vi "Add File Name on PDF.vi"(11 "error in (no error)":errorcluster) -> (6 "Path":path, 15 "error out":errorcluster)   [LabVIEW 2019]
doc: "Location: at the end of the report generation.\n\nThis can only be followed by \"Print PDF.vi\" and \"Dispose references.vi\".\n\nVersion 1.0\nDeveloped by Jean-Marc Simard\nCopyright © 2010, Exaprom Inc.\nAll rights reserved.\nLicense: BSD\n\nWith iTextSharp Library\n(http://itextsharp.sourceforge.net)"
uses:
  <userlib>/Exaprom PDF/LV Class/Header and Footer Class/VIs/Controls/Header Footer [ ] V2.ctl
  <userlib>/Exaprom PDF/LV Class/Header and Footer Class/VIs/Controls/Header Footer cluster V2.ctl
  <userlib>/Exaprom PDF/Controls/Header, Footer and Watermark Controls/Header or Footer.ctl
  <userlib>/Exaprom PDF/Controls/Header, Footer and Watermark Controls/Header Footer Type.ctl
  <userlib>/Exaprom PDF/Controls/Header, Footer and Watermark Controls/Header footer horiz alignment.ctl
  <userlib>/Exaprom PDF/Controls/Table Controls/Cell Vertical alignment.ctl
  <userlib>/Exaprom PDF/Controls/Text Controls/Line spacing.ctl
  <userlib>/Exaprom PDF/Controls/Header, Footer and Watermark Controls/Page number.ctl
  <userlib>/Exaprom PDF/Controls/Font Controls/Font complete cluster horizontal.ctl
  <userlib>/Exaprom PDF/Controls/Font Controls/Font size.ctl
  <userlib>/Exaprom PDF/Controls/Font Controls/Font color.ctl
  <userlib>/Exaprom PDF/Controls/Font Controls/Type and encoding.ctl
  <userlib>/Exaprom PDF/Controls/Text Controls/Unicode/Type and run direction.ctl
  C:/Program Files/National Instruments/LabVIEW 2019/user.lib/Exaprom PDF/DLL/itextsharp.dll
  DLL/itextsharp.dll
  <userlib>/Exaprom PDF/Controls/Header, Footer and Watermark Controls/Header Footer Line.ctl
  <userlib>/Exaprom PDF/Controls/Page Controls/Page dimensions.ctl
  <userlib>/Exaprom PDF/Controls/Page Controls/Page size.ctl
  <userlib>/Exaprom PDF/Controls/Page Controls/Page Orientation.ctl
panel:
  in  "Header or Footer [ ]":T1
  in  "Path 2":path
  # "X"
  # "Y"
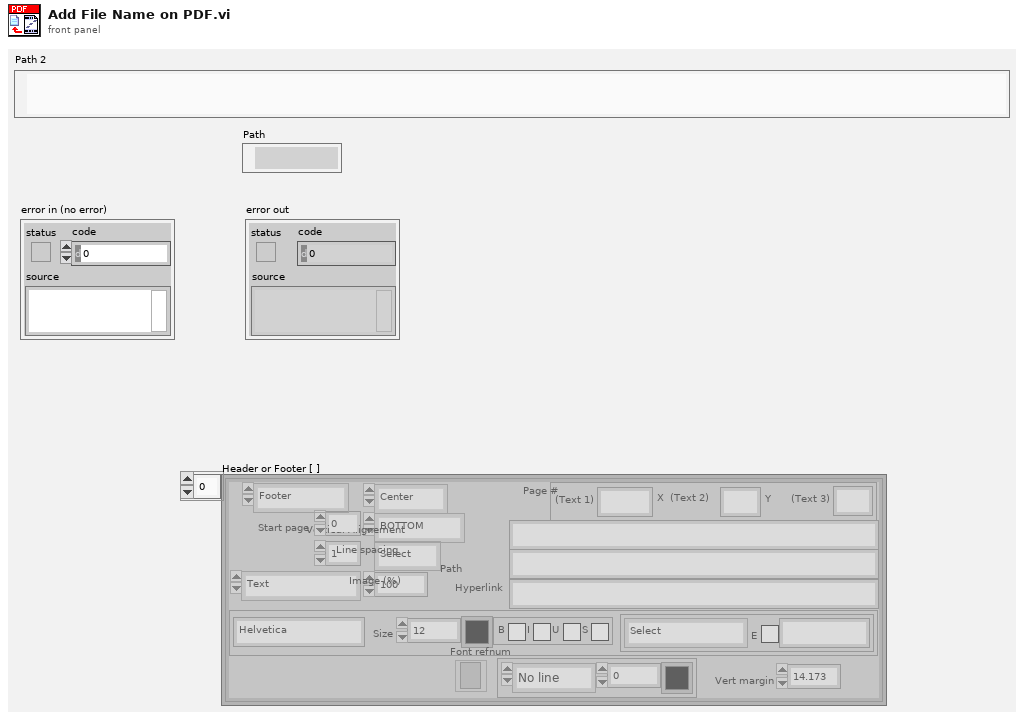
[diagram p1: front panel]
types:
  T1 = typedef "Header Footer [ ] V2.ctl" = T2[]
  T2 = typedef "Header Footer cluster V2.ctl" = cluster{"Header or Footer":T3, "Start page":i32, "Start with #":i32, "Type":T4, "Alignment":T5, "Vertical Alignement":T6, "Line spacing":T7, "Image (%)":sgl, "Page #":T8, "Text":string, "Path":string, "Font":T9, "Font refnum":refnum<k24>, "Line":cluster{"Line":T14, "Thickness (points)":sgl, "Colour":T11}, "Vert margin":dbl, "Hyperlink":string}
  T3 = typedef "Header or Footer.ctl" = enum16{"Header", "Footer"}
  T4 = typedef "Header Footer Type.ctl" = enum16{"Select", "Text", "Text + hyperlink", "Page number", "Image", "Image + hyperlink"}
  T5 = typedef "Header footer horiz alignment.ctl" = enum16{"Left", "Center", "Right"}
  T6 = typedef "Cell Vertical alignment.ctl" = enum16{"TOP", "MIDDLE", "BOTTOM"}
  T7 = typedef "Line spacing.ctl" = enum16{"Select", "1.0", "1.5", "2.0"}
  T8 = typedef "Page number.ctl" = cluster{"Text 1":string, "Text 2":string, "Text 3":string}
  T9 = typedef "Font complete cluster horizontal.ctl" = cluster{"Name":string, "Size":T10, "Color":T11, "Style":cluster{"Bold":bool, "Italic":bool, "Underline":bool, "Strikeout":bool}, "Type":T12}
  T10 = typedef "Font size.ctl" = sgl
  T11 = typedef "Font color.ctl" = u32
  T12 = typedef "Type and encoding.ctl" = cluster{"Type&direction":T13, "Embedded":bool, "Encoding":string}
  T13 = typedef "Type and run direction.ctl" = enum16{"Select", "ASCII", "UTF-16", "UTF-16 (default)", "UTF-16 (LTR)", "UTF-16 (RTL)"}
  T14 = typedef "Header Footer Line.ctl" = enum16{"No line", "Horizontal line"}
  T15 = typedef "Page dimensions.ctl" = cluster{"Start at page":i32, "Page Size":T16, "Orientation":T17, "widht":sgl, "height":sgl, "Margin left":sgl, "Margin right":sgl, "Margin top":sgl, "Margin bottom":sgl, "X0":sgl, "X1":sgl, "Y0":sgl, "Y1":sgl}
  T16 = typedef "Page size.ctl" = i32
  T17 = typedef "Page Orientation.ctl" = enum16{"Portrait", "Landscape"}
  T18 = typedef "Header Footer Complete Cluster.ctl" = cluster{"Table position":T19, "Header Footer Cluster with references [ ]":T20[]}
  T19 = typedef "Header or Footer Position.ctl" = cluster{"Vert margin":dbl, "FixedHeight":dbl, "Table X postion":dbl, "Table Y postion":dbl}
  T20 = typedef "Header Footer Cluster with references.ctl" = cluster{"Start page":i32, "Type":T4, "Start with #":i32, "Alignment":T5, "Vertical Alignement":T6, "Page #":T8, "Text":refnum<k24>, "Scaled Img":refnum<k24>, "PdfPCell":refnum<k24>, "PdfPTable":refnum<k24>, "Font Cluster":T9, "Font ":refnum<k24>, "Img (%)":sgl, "Line":cluster{"Line":T14, "Thickness (points)":sgl, "Colour":T11}, "Line spacing":T7}
  T21 = typedef "Watermark cluster2.ctl" = cluster{"Show? (F)":bool, "Type":enum16{"Image", "Text"}, "Opacity (%)":sgl, "Rotate(°)":sgl, "Position":cluster{"Position":T22, "X":sgl, "Y":sgl}, "Image path":path, "Scaled(%)":sgl, "Image refnum":refnum<k24>, "Text":string, "Font":cluster{"Name":string, "Size":T10, "Color":T11}, "Font refnum":refnum<k24>, "Alignment":T5, "Automatic":bool}
  T22 = typedef "Watermark Position.ctl" = enum16{"Absolute", "Center (page)", "Center (text section)"}
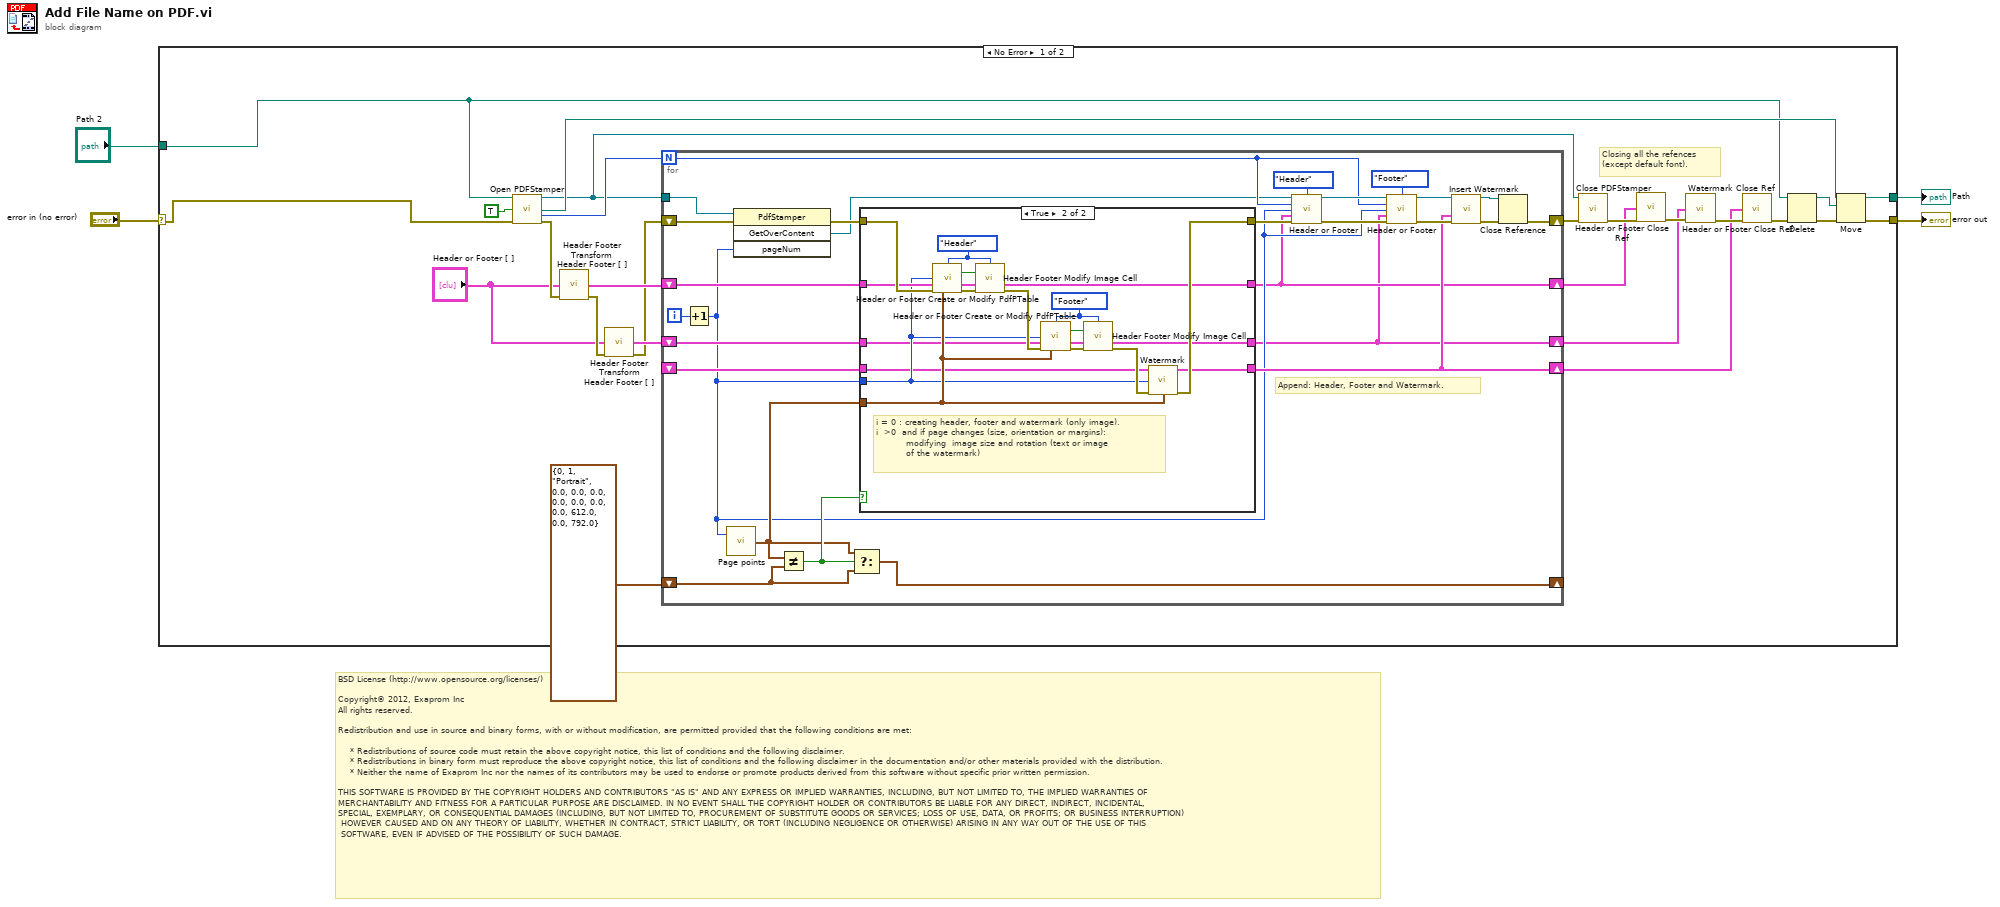
[diagram p0: block diagram]
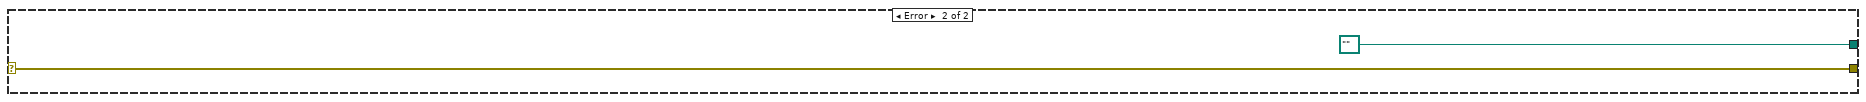
[diagram p3: hidden frame]
diagram:
  # "BSD License (http://www.opensource.org/licenses/)\n\nCopyright© 2012, Exaprom Inc\nAll rights reserved.\n\nRedistribution and use in source and binary forms, with or without modification, are permitted provided that the following conditions are met:\n\n    * Redistributions of source code must retain the above copyright notice, this list of conditions and the following disclaimer.\n    * Redistributions in binary form must reproduce the above copyright notice, this list of conditions and the following disclaimer in the documentation and/or other materials provided with the distribution.\n    * Neither the name of Exaprom Inc nor the names of its contributors may be used to endorse or promote products derived from this software without specific prior written permission.\n\nTHIS SOFTWARE IS PROVIDED BY THE COPYRIGHT HOLDERS AND CONTRIBUTORS \"AS IS\" AND ANY EXPRESS OR IMPLIED WARRANTIES, INCLUDING, BUT NOT LIMITED TO, THE IMPLIED WARRANTIES OF \nMERCHANTABILITY AND FITNESS FOR A PARTICULAR PURPOSE ARE DISCLAIMED. IN NO EVENT SHALL THE COPYRIGHT HOLDER OR CONTRIBUTORS BE LIABLE FOR ANY DIRECT, INDIRECT, INCIDENTAL,\nSPECIAL, EXEMPLARY, OR CONSEQUENTIAL DAMAGES (INCLUDING, BUT NOT LIMITED TO, PROCUREMENT OF SUBSTITUTE GOODS OR SERVICES; LOSS OF USE, DATA, OR PROFITS; OR BUSINESS INTERRUPTION)\n HOWEVER CAUSED AND ON ANY THEORY OF LIABILITY, WHETHER IN CONTRACT, STRICT LIABILITY, OR TORT (INCLUDING NEGLIGENCE OR OTHERWISE) ARISING IN ANY WAY OUT OF THE USE OF THIS\n SOFTWARE, EVEN IF ADVISED OF THE POSSIBILITY OF SUCH DAMAGE."
  n1 = case shown="No Error" "error in (no error)" {
    selector: "error in (no error)" -> [w6 w82]
    tunnel: [w8 w82] -> w4
    tunnel: [w29 path "" ("new path")] -> w2
    tunnel: "Path 2" -> [w7 _]
    frame No Error {
      # "Closing all the refences \n(except default font)."
      n2 = call <userlib>:"Open PDFStamper.vi"("PDF Path (original)"=w7, "RotateContents (F)"=TRUE, "error in (no error)"=w6) -> ("PDFStamper"=w19:refnum<k24>, "Temporary File Name"=w25:path, "NumberOfPages"=w27:i32, "error out"=w15:errorcluster)  [unwired: 4 in, 5 out]
      n3 = call <userlib>:"Header Footer Transform Header Footer [ ].vi"("Header or Footer [ ]"="Header or Footer [ ]", "error in (no error)"=w15) -> ("Header or Footer Complete Cluster"=w18:T18, "error out"=w16:errorcluster)  [unwired: 12 out]
      n4 = call <userlib>:"Header Footer Transform Header Footer [ ].vi"("Header or Footer [ ]"="Header or Footer [ ]", "error in (no error)"=w16) -> ("Header or Footer Complete Cluster"=w17:T18, "error out"=w14:errorcluster)  [unwired: 12 out]
      n5 = for {
        N: w27 -> [w45]
        tunnel: w19 -> [w50]
        shift-right: [w44] -> _
        shift-left: T15 {"Start at page"=0, "Page Size"=1, "Orientation"=enum."Portrait", "widht"=0.0, "height"=0.0, "Margin left"=0.0, "Margin right"=0.0, "Margin top"=0.0, "Margin bottom"=0.0, "X0"=0.0, "X1"=612.0, "Y0"=0.0, "Y1"=792.0} ("Page (points)") -> [w43]
        shift-right: [w38] -> w9
        shift-left: _ -> [w37]
        shift-right: [w36] -> w26
        shift-left: w14 -> [w51]
        shift-right: [w32] -> w13
        shift-left: w18 -> [w41]
        shift-right: [w31] -> w12
        shift-left: w17 -> [w39]
        i -> [w52]
        # "Append: Header, Footer and Watermark."
        n6 = Increment(x=w52) -> (x+1=w33:i32)
        n7 = call <userlib>:"Page points.vi"("pageNum"=w33) -> ("Page (points)"=w40:T15)  [unwired: 1 in]
        n8 = invoke class="PdfStamper" method="GetOverContent"(reference=w50, error in=w51, "pageNum"=w33) -> (error out=w55:errorcluster, "GetOverContent"=w30:refnum<k24>)  [unwired: 1 in, 2 out]
        n9 = Not Equal?(x=w40, y=w43) -> (x != y?=w42:bool)
        n10 = Select(t=w40, s=w42, f=w43) -> (s? t:f=w44:T15)
        n11 = case shown="True" w42 {
          tunnel: w41 -> [w59 w76]
          tunnel: w40 -> [_ w72]
          tunnel: w39 -> [w58 w63]
          tunnel: w55 -> [w57 w80]
          tunnel: [w57 w78] -> w56
          tunnel: w37 -> [w60 w68]
          tunnel: [w60 w73] -> w38
          tunnel: w33 -> [_ w71]
          tunnel: [w59 w65] -> w32
          tunnel: [w58 w64] -> w31
          frame False {
          }
          frame True {
            w69 = Header_or_Footer."Footer" ("Header or Footer")
            w70 = Header_or_Footer."Header" ("Header or Footer")
            # "i = 0 : creating header, footer and watermark (only image).\ni  >0  and if page changes (size, orientation or margins):\n          modifying  image size and rotation (text or image \n          of the watermark)"
            n12 = call <userlib>:"Header or Footer Create or Modify PdfPTable.vi"("Header or Footer"=w70, "pageNum"=w71, "Header Footer IN [ ]"=w76, "error in (no error)"=w80, "Page points"=w72) -> ("Modify Image Cell"=w62:bool, "Header Footer OUT [ ]"=w66:T18, "error out"=w75:errorcluster)  [unwired: 3 in, 5 out]
            n13 = call <userlib>:"Header Footer Modify Image Cell.vi"("Header or Footer"=w70, "Modify Image Cell"=w62, "Header or Footer Complete Cluster IN"=w66, "error in (no error)"=w75) -> ("Header or Footer Complete Cluster OUT"=w65:T18, "error out"=w77:errorcluster)  [unwired: 1 in, 9 out]
            n14 = call <userlib>:"Header or Footer Create or Modify PdfPTable.vi"("Header or Footer"=w69, "pageNum"=w71, "Header Footer IN [ ]"=w63, "error in (no error)"=w77, "Page points"=w72) -> ("Modify Image Cell"=w61:bool, "Header Footer OUT [ ]"=w67:T18, "error out"=w74:errorcluster)  [unwired: 3 in, 5 out]
            n15 = call <userlib>:"Header Footer Modify Image Cell.vi"("Header or Footer"=w69, "Modify Image Cell"=w61, "Header or Footer Complete Cluster IN"=w67, "error in (no error)"=w74) -> ("Header or Footer Complete Cluster OUT"=w64:T18, "error out"=w79:errorcluster)  [unwired: 1 in, 9 out]
            n16 = call <userlib>:"Watermark.vi"("Watermark IN"=w68, "pageNum"=w71, "error in (no error)"=w79, "Page dimensions"=w72) -> ("Watermark OUT"=w73:T21, "error out"=w78:errorcluster)  [unwired: 2 in, 8 out]
          }
        }
        n17 = call <userlib>:"Header or Footer.vi"("OverContent"=w30, "Header or Footer"=Header_or_Footer."Header", "NumberOfPages"=w45, "pageNum"=w33, "Header or Footer Complete Cluster"=w32, "error in (no error)"=w56) -> ("OverContent duplicate"=w53:refnum<k24>, "error out"=w54:errorcluster)  [unwired: 2 in, 6 out]
        n18 = call <userlib>:"Header or Footer.vi"("OverContent"=w53, "Header or Footer"=Header_or_Footer."Footer", "NumberOfPages"=w45, "pageNum"=w33, "Header or Footer Complete Cluster"=w31, "error in (no error)"=w54) -> ("OverContent duplicate"=w48:refnum<k24>, "error out"=w49:errorcluster)  [unwired: 1 in, 7 out]
        n19 = call <userlib>:"Insert Watermark.vi"("OverContent"=w48, "Watermark Cluster"=w38, "error in (no error)"=w49) -> ("OverContent duplicate"=w46:refnum<k24>, "error out"=w47:errorcluster)  [unwired: 3 in, 8 out]
        n20 = Close Reference(reference=w46, error in (no error)=w47) -> (error out=w36:errorcluster)
      }
      n21 = call <userlib>:"Close PDFStamper.vi"("PDFStamper"=w19, "error in (no error)"=w26) -> ("error out"=w21:errorcluster)  [unwired: 13 out]
      n22 = call <userlib>:"Header or Footer Close Ref.vi"("Header or Footer Complete Cluster"=w13, "error in (no error)"=w21) -> ("error out"=w20:errorcluster)  [unwired: 2 in, 11 out]
      n23 = call <userlib>:"Header or Footer Close Ref.vi"("Header or Footer Complete Cluster"=w12, "error in (no error)"=w20) -> ("error out"=w11:errorcluster)  [unwired: 1 in, 12 out]
      n24 = call <userlib>:"Watermark Close Ref.vi"("Watermark IN"=w9, "error in (no error)"=w11) -> ("error out"=w10:errorcluster)  [unwired: 1 in, 12 out]
      n25 = Delete(path (use dialog)=w7, error in=w10) -> (deleted path=w23:path, error out=w22:errorcluster)  [unwired: 4 out]
      n26 = Move(source path=w25, error in=w22, 10:w23) -> (error out=w8:errorcluster, 3:w29:path)  [unwired: 3 out]
    }
    frame Error {
    }
  }
  "error out" <- w4
  "Path" <- w2
